vi "Main_11B_X1.vi"() -> ()   [LabVIEW 2024]
panel:
  in  "Example 2":string="125 17"
  in  "Use Puzzle":bool
  out "Answer 191690":u32
  in  "Puzzle":string="30 71441 3784 580926 2 8122942 0 291"
  in  "Example":string="0 1 10 99 999"
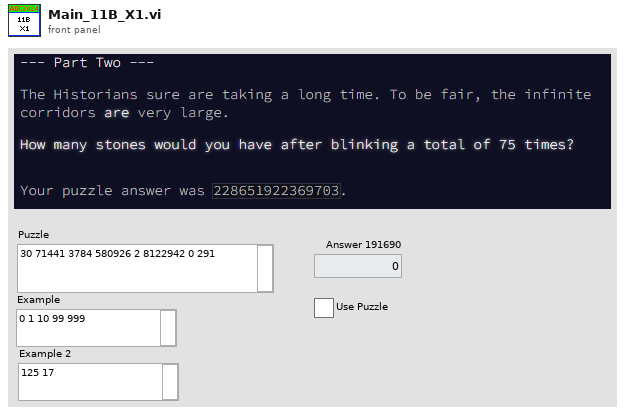
[diagram p1: front panel]
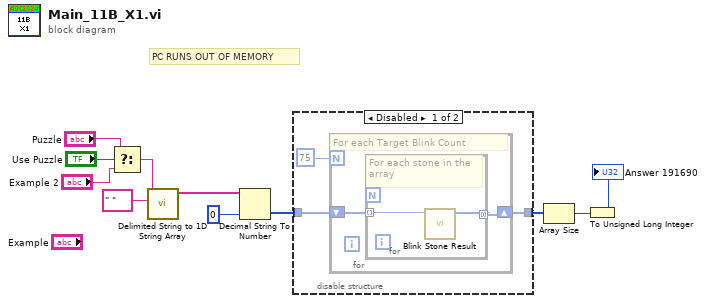
[diagram p0: block diagram]
diagram:
  # "PC RUNS OUT OF MEMORY"
  n1 = Select(t="Puzzle", s="Use Puzzle", f="Example 2") -> (s? t:f=w9:string)
  n2 = call <vilib>:"Delimited String to 1D String Array.vi"("delimiter"=" " ("delimiter (Tab)"), "delimited string"=w9) -> ("string array"=w10:string[])  [unwired: 9 in]
  n3 = Decimal String To Number(string=w10, default (0L)=u64 0 ("default (0 I32)")) -> (number=w5:u64[])  [unwired: 1 in, 1 out]
  n4 = disable-structure shown="Disabled" {
    disable-tunnel: w5 -> [w14 _]
    disable-tunnel: [w12 _] -> w1
    frame Disabled {
      n5 = for {
        N: 75 -> [_]
        shift-right: [w16] -> w12
        shift-left: w14 -> [w15]
        # "For each Target Blink Count"
        n6 = for {
          tunnel: w15 -> [w18] mode=indexing
          tunnel: [w17] -> w16 mode=concatenating
          # "For each stone in the array"
          n7 = call "Blink Stone Result.vi"("String"=w18) -> ("Result Array"=w17:u64[])  [unwired: 9 in, 1 out]
        }
      }
    }
    frame Enabled {
    }
  }
  n8 = Array Size(array=w1) -> (size(s)=w3:i32)
  n9 = To Unsigned Long Integer(number=w3) -> (unsigned 32bit integer=→"Answer 191690":u32)
